vi "Configure UI Component.vi"(10 "SubPanel Reference":refnum<vi>, 11 "Base UI Component in":refnum<class "Base UI Component.lvclass">) -> (3 "Base UI Component out":refnum<class "Base UI Component.lvclass">)   [LabVIEW 2016, in "Assert Display.lvlib" / "Base UI Component.lvlib" / "Base UI Component.lvclass"]
uses:
  Base UI Component.lvclass
  Base UI Component.lvclass/Base UI Component.ctl
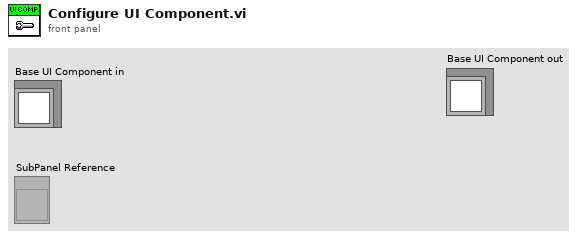
[diagram p1: front panel]
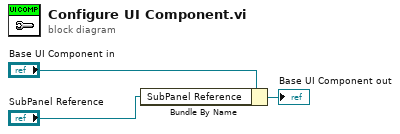
[diagram p0: block diagram]
diagram:
  n1 = Bundle By Name(cluster="Base UI Component in", "SubPanel Reference"="SubPanel Reference") -> (→"Base UI Component out":refnum<class "Base UI Component.lvclass">)
